vi "BooleanAsValue.vi"(8 "error in":errorcluster, 11 "scalar value (boolean)":bool) -> (0 "error out":errorcluster, 3 "scalar string":string)   [LabVIEW 2014]
doc: "Format a LV boolean as an XML-RPC boolean type"
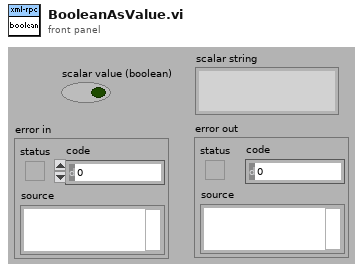
[diagram p1: front panel]
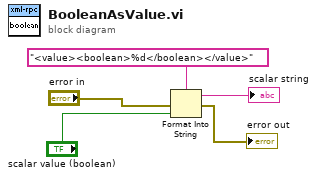
[diagram p0: block diagram]
diagram:
  n1 = Format Into String(format string="<value><boolean>%d</boolean></value>", error in="error in", "scalar value (boolean)") -> (resulting string=→"scalar string":string, error out=→"error out":errorcluster)  [unwired: 1 in]
